vi "Create_Simple_Var.vi"(4 "Value":T1) -> (1 "Var":refnum<class "Var_Bool.lvclass">)   [LabVIEW 2021, in "Var_Bool.lvclass"]
uses:
  Var_Bool.lvclass
  Type.ctl
  Var_Bool.lvclass/Var_Bool.ctl
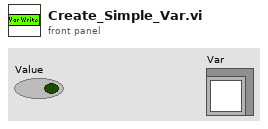
[diagram p1: front panel]
types:
  T1 = typedef "Var_Bool.lvclass/Type.ctl" = bool
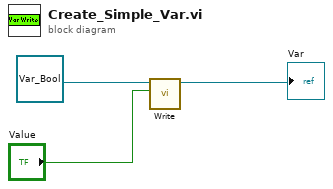
[diagram p0: block diagram]
diagram:
  n1 = call-dynamic "Write.vi"("Value"="Value", "Double Float.lvclass_340760 in"=refnum<class "Var_Bool.lvclass"> refnum ("Constants.lvlib:Numeric.lvclass")) -> ("Double Float.lvclass_340760 out"=→"Var":refnum<class "Var_Bool.lvclass">)  [unwired: 8 in, 1 out]
